vi "SH_ComputeFitness.vi"(8 "error in (no error)":errorcluster, 9 "Notifier":refnum<notifier>, 10 "Shapelets Queue":refnum<queue>, 11 "ShapeletClass in":refnum<class "Shapelets Search Brute Force.lvclass">) -> (0 "error out":errorcluster, 2 "Fitness Values":dbl[](array[numeric]), 3 "ShapeletClass out":refnum<class "Shapelets Search Brute Force.lvclass">)   [LabVIEW 2016, in "Shapelets Search (Brute Force).lvlib" / "Shapelets Search Brute Force.lvclass"]
uses:
  Shapelets Search Brute Force.lvclass
  SH_Shapelet.ctl
  Shapelets Search Brute Force.lvclass/Shapelets Search Brute Force.ctl
  <vilib>/Analysis/baseanly.llb/Normalize Vector.vi
  Shapelets Search (Brute Force).lvlib
  <vilib>/Analysis/NI_AALPro.lvlib
  <vilib>/Analysis/NI_AALBase.lvlib
panel:
  # "This VI is a part of BCI Design library, http://www.ru-bci.org \nCopyright © 2020, Sotnikov Peter, All rights reserved. License: GNU GPLv3"
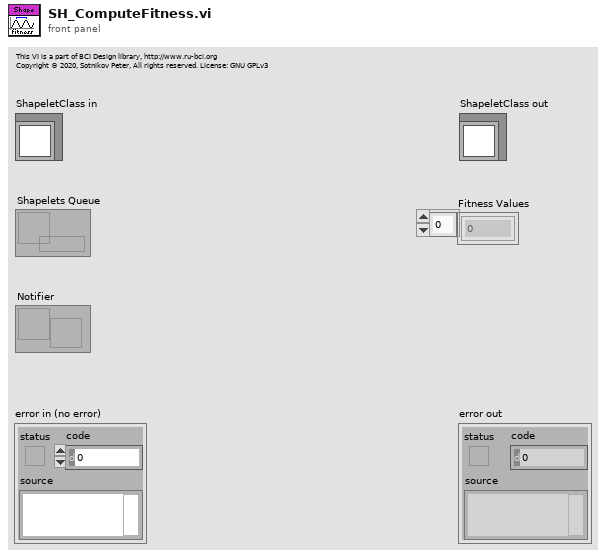
[diagram p1: front panel]
types:
  T1 = cluster{"ClassLabel":string, "FeatureVector":dbl[][]}[]
  T2 = typedef "Shapelets Search (Brute Force).lvlib/SH_Shapelet.ctl" = cluster{"TrialIndex":i32, "Shift (in samples)":i32, "Length (in samples)":i32, "Distances":dbl[], "ClassIndecies":i32[], "Fitness":dbl, "Split Point":dbl}
  T3 = cluster{"ClassLabel":string, "FeatureVector":dbl[][]}
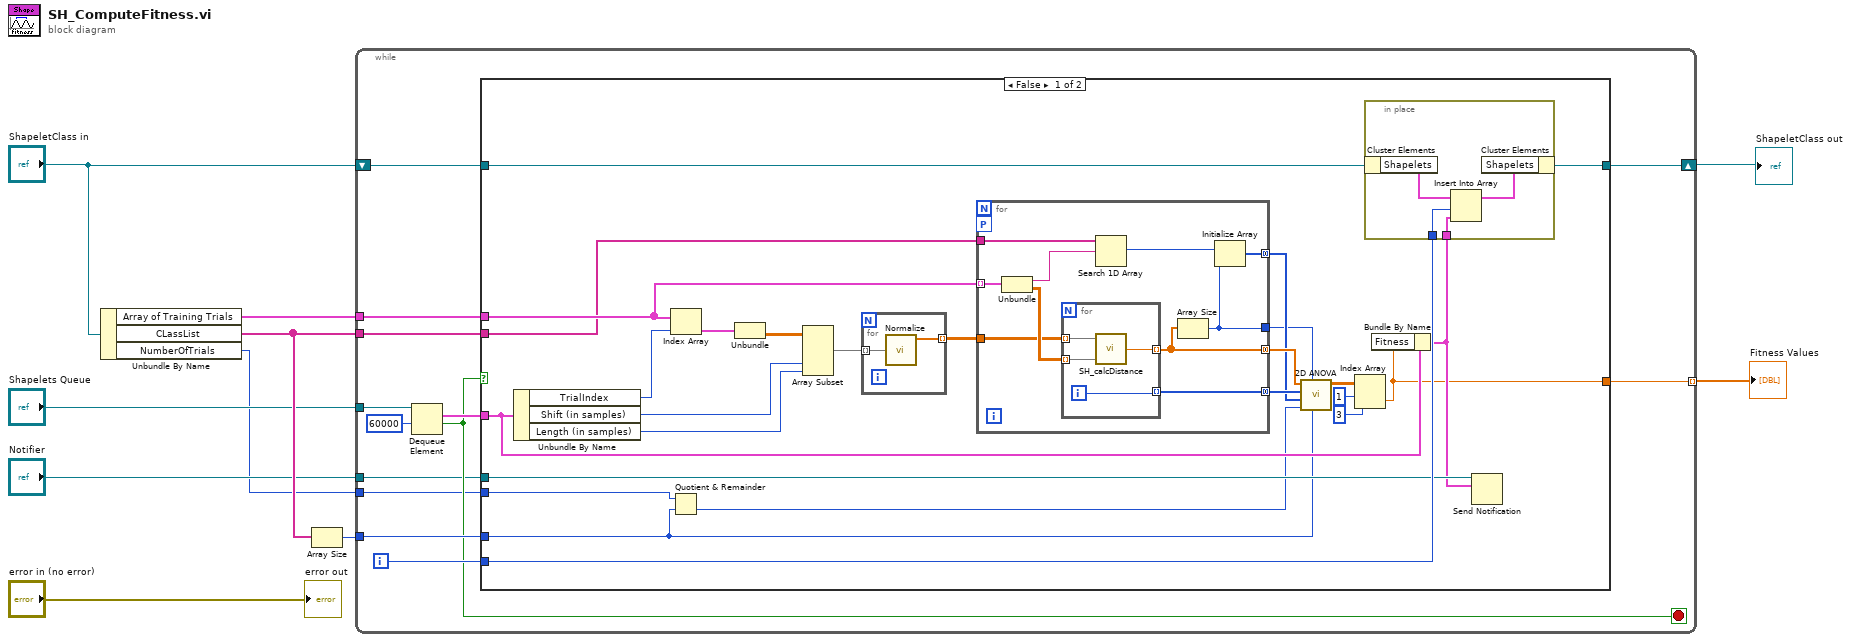
[diagram p0: block diagram]
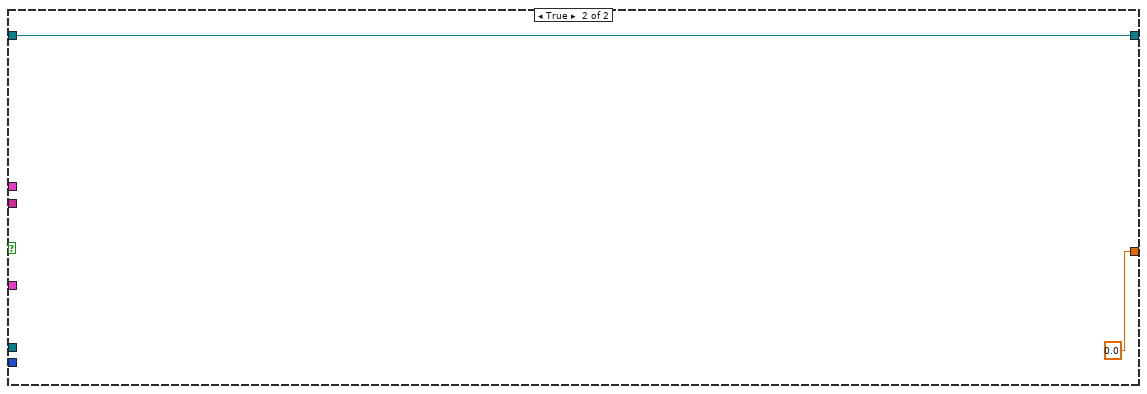
[diagram p2: hidden frame]
diagram:
  n1 = Unbundle By Name("ShapeletClass in") -> ("Array of Training Trials"=w10:T1, "CLassList"=w5:string[], "NumberOfTrials"=w1:i32)
  n2 = Array Size(array=w5) -> (size(s)=w6:i32)
  n3 = while {
    tunnel: w10 -> [w23]
    tunnel: w5 -> [w22]
    shift-right: [w20] -> w8
    shift-left: "ShapeletClass in" -> [w21]
    tunnel: w6 -> [w19]
    tunnel: [w17] -> w4 mode=indexing
    tunnel: "Shapelets Queue" -> [w16]
    tunnel: "Notifier" -> [w12]
    tunnel: w1 -> [w11]
    i -> [w18]
    stop <- w13 stop-if-true
    n4 = Dequeue Element(queue=w16, timeout in ms (-1)=60000) -> (element=w15:T2, timed out?=w13:bool)  [unwired: 1 in, 2 out]
    n5 = case shown="False" w13 {
      tunnel: w23 -> [w46 _]
      tunnel: w22 -> [w45 _]
      tunnel: w21 -> [w43 w71]
      tunnel: [w42 w71] -> w20
      tunnel: w19 -> [w29 _]
      tunnel: w18 -> [w41 _]
      tunnel: [w26 0.0 ("f")] -> w17
      tunnel: w15 -> [w40 _]
      tunnel: w12 -> [w39 _]
      tunnel: w11 -> [w30 _]
      frame False {
        n6 = Unbundle By Name(w40) -> ("TrialIndex"=w49:i32, "Shift (in samples)"=w36:i32, "Length (in samples)"=w37:i32)
        n7 = Index Array(array=w46, index=w49) -> (element=w48:T3)
        n8 = Quotient & Remainder(x=w30, y=w29) -> (floor(x/y)=w28:i32)  [unwired: 1 out]
        n9 = Unbundle(w48) -> ("FeatureVector"=w47:dbl[][])  [unwired: 1 out]
        n10 = Array Subset(array=w47, index (col)=w36, length (col)=w37) -> (w35:dbl[][])  [unwired: 2 in]
        n11 = for {
          tunnel: [w51] -> w44 mode=indexing
          tunnel: w35 -> [w50] mode=indexing
          n12 = call-poly <vilib>:"Normalize.vi"("Vector"=w50) -> ("Normalized Vector"=w51:dbl[])  [unwired: 1 in, 3 out]
        }
        n13 = for {
          tunnel: w46 -> [w65] mode=indexing
          tunnel: w45 -> [w64]
          tunnel: w44 -> [w61]
          workers-P: _ -> [_]
          tunnel: [w59] -> w34 mode=concatenating
          tunnel: [w60] -> w33 mode=concatenating
          tunnel: [w57] -> w32 mode=concatenating
          tunnel: [w56] -> w31
          n14 = Unbundle(w65) -> ("ClassLabel"=w63:string, "FeatureVector"=w62:dbl[][])
          n15 = for {
            tunnel: w62 -> [w68] mode=indexing
            tunnel: w61 -> [w69] mode=indexing
            tunnel: [w67] -> w59 mode=indexing
            tunnel: [w66] -> w60 mode=indexing
            i -> [w66]
            n16 = call "SH_calcDistance.vi"("Time series"=w68, "Shapelet (normalized)"=w69) -> ("Distance out"=w67:dbl)  [unwired: 1 in]
          }
          n17 = Search 1D Array(1D array=w64, element=w63) -> (index of element=w58:i32)  [unwired: 1 in]
          n18 = Array Size(array=w59) -> (size(s)=w56:i32)
          n19 = Initialize Array(w58, w56) -> (w57:i32[])
        }
        n20 = call <vilib>:"2D ANOVA.vi"("B levels"=w29, "A levels"=w31, "observations per cell"=w28, "Index B"=w32, "Index A"=w33, "X"=w34) -> ("Info"=w27:dbl[][])  [unwired: 1 in, 4 out]
        n21 = Index Array(array=w27, index (row)=1, index (col)=3 ("disabled index (col)")) -> (element=w26:dbl)
        n22 = Bundle By Name(cluster=w40, "Fitness"=w26) -> (w38:T2)
        n23 = in-place {
          in-place-border: w41 -> [w53]
          in-place-border: w38 -> [w52]
          n24 = in-place-cluster #1(w43) -> ("Shapelets"=w55:T2[])
          n25 = Insert Into Array(array=w55, index=w53, new element=w52) -> (w54:T2[])
          n26 = in-place-cluster #1("Shapelets"=w54) -> (w42:refnum<class "Shapelets Search Brute Force.lvclass">)
        }
        n27 = Send Notification(notification=w38, notifier=w39) -> ()  [unwired: 1 in, 2 out]
      }
      frame True {
      }
    }
  }
  "ShapeletClass out" <- w8
  "Fitness Values" <- w4
  "error out" <- "error in (no error)"
